vi "traffic control monitor.vi"(8 "error in (no error)":errorcluster, 10 "remote port or service name":u16=4001, 11 "address":string="212.169.106.189") -> (0 "error out":errorcluster, 1 "RMAD Signalys Monitor":T1 {"Uptime  (W:D:H)" format="%<%W:%D:%H>t"}, 2 "up time (W:D:H:M:S)":dbl format="%<%W:%D:%H:%M:%S>t", 3 "RMAD signallys STATUS":bool)   [LabVIEW 2017]
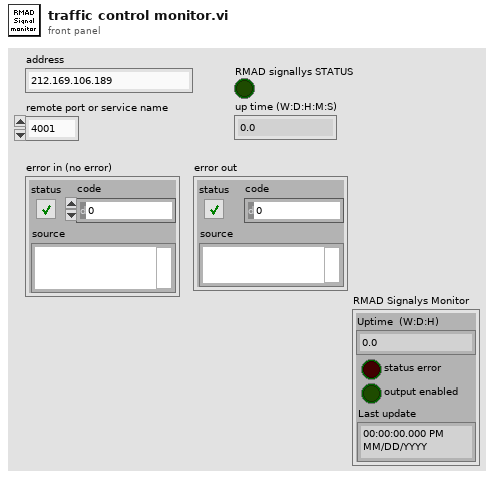
[diagram p1: front panel]
types:
  T1 = cluster{"Uptime  (W:D:H)":dbl, "status error":bool, "output enabled":bool, "Last update":timestamp}
  T2 = enum16{"Standard", "Buffered", "CRLF", "Immediate"}
  T3 = cluster{dbl, bool, bool, "seconds since 1Jan1904":timestamp}
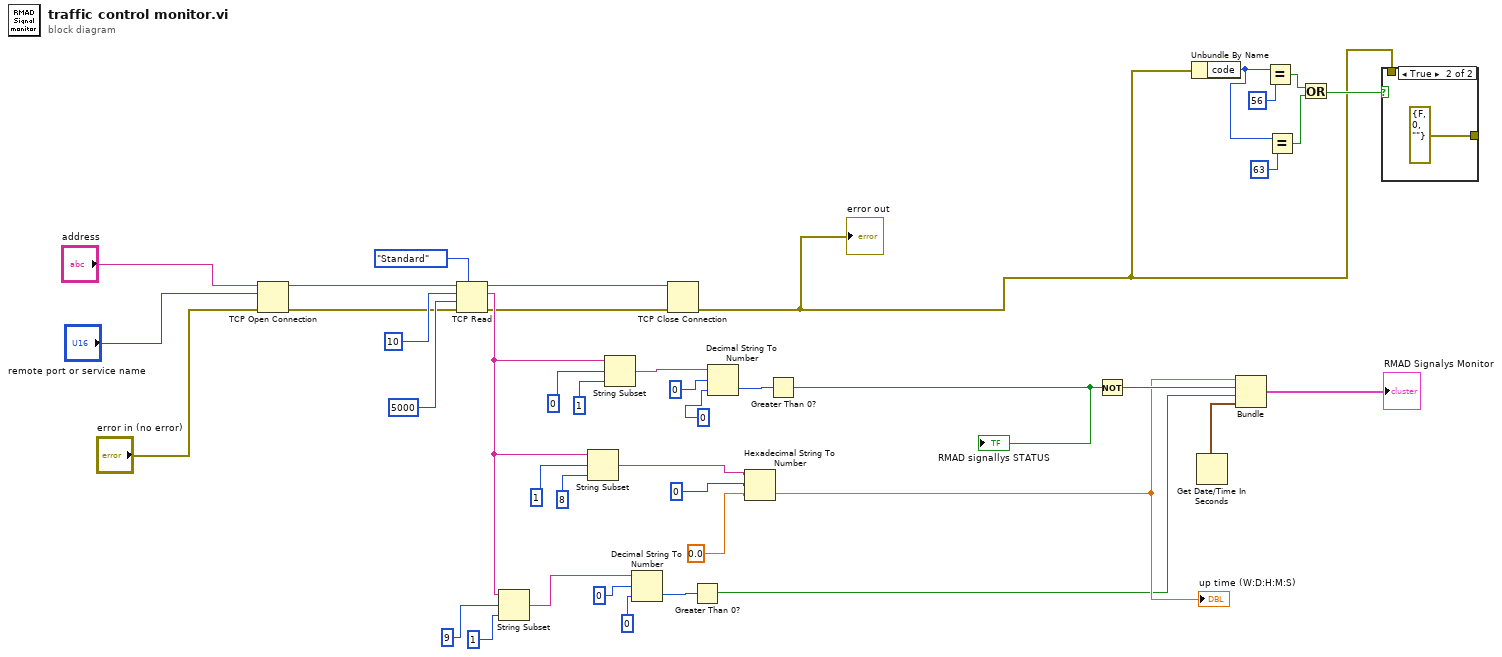
[diagram p0: block diagram]
diagram:
  n1 = TCP Open Connection(address="address", remote port or service name="remote port or service name", error in (no error)="error in (no error)") -> (connection ID=w35:refnum<k5>, error out=w36:errorcluster)  [unwired: 2 in]
  n2 = TCP Read(connection ID=w35, bytes to read=10, error in (no error)=w36, 7:T2."Standard" ("mode (standard)"), 9:5000 ("timeout ms (25000)")) -> (connection ID out=w34:refnum<k5>, data out=w19:string, error out=w15:errorcluster)
  n3 = String Subset(string=w19, offset (0)=9, length (rest)=1 ("length (rest)")) -> (substring=w14:string)
  n4 = String Subset(string=w19, offset (0)=1, length (rest)=8 ("length (rest)")) -> (substring=w25:string)
  n5 = String Subset(string=w19, offset (0)=0, length (rest)=1 ("length (rest)")) -> (substring=w28:string)
  n6 = Decimal String To Number(string=w14, offset=0, default (0L)=u8 0) -> (number=w13:u8)  [unwired: 1 out]
  n7 = TCP Close Connection(connection ID=w34, error in (no error)=w15) -> (error out=w1:errorcluster)  [unwired: 1 in, 1 out]
  "error out" <- w1
  n8 = Greater Than 0?(x=w13) -> (x > 0?=w8:bool)
  n9 = Decimal String To Number(string=w28, offset=0, default (0L)=u8 0) -> (number=w29:u8)  [unwired: 1 out]
  n10 = Hexadecimal String To Number(string=w25, offset=0, default (0uL)=0.0 ("up time (W:D:H) 2")) -> (number=w18:dbl)  [unwired: 1 out]
  "up time (W:D:H:M:S)" <- w18
  n11 = Greater Than 0?(x=w29) -> (x > 0?=w20:bool)
  "RMAD signallys STATUS" <- w20
  n12 = Not(x=w20) -> (.not. x?=w21:bool)
  n13 = Unbundle By Name(w1) -> ("code"=w7:i32)
  n14 = Get Date/Time In Seconds() -> (seconds since 1Jan1904=w17:timestamp)
  n15 = Bundle(w18, w21, w8, "seconds since 1Jan1904"=w17) -> (→"RMAD Signalys Monitor":T3)  [unwired: 1 in]
  n16 = Equal?(x=w7, y=56) -> (x = y?=w4:bool)
  n17 = Equal?(x=w7, y=63) -> (x = y?=w5:bool)
  n18 = Or(x=w4, y=w5) -> (x .or. y?=w6:bool)
  n19 = case shown="True" w6 {
    tunnel: [w42 errorcluster {"status"=FALSE, "code"=0, "source"=""} ("error out")] -> _
    tunnel: w1 -> [w42 _]
    frame False {
    }
    frame True {
    }
  }
